vi "ColorTracking_lab.vi"(0 "ROI Descriptor (Color Location 1)":T2={"Global Rectangle"=[20, 20, 620, 460], "Contours"=[{"ID"=enum."External", "Type"=12, "Coordinates"=[20, 20, 620, 460, 0]}]} {"Contours"."Type" items=["No Selection", "Point", "Line", "Rectangle", "Oval", "Polygon", "Freehand Region", "Annulus", "Unused2", "Unused3", "Broken Line", "Freehand Line", "Rotated Rectangle"]}, 1 "File Path (Color Location 1)":path=path "C:/Users/canlasd/Downloads/Labview/Templates/T1.png", 2 "Minimum Match Score (Color Location 1)":sgl=500.0) -> (20 "Matches (Color Location 1)":T3(array[cluster]) {"Bounding Box"."y" format="%.2f"; "Bounding Box"."x" format="%.2f"; "Position"."y" format="%.2f"; "Position"."x" format="%.2f"; "Score" format="%.2f"; "Scale" format="%.2f"; "Angle" format="%.2f"}, 21 "Matches (calibrated) (Color Location 1)":T3(array[cluster]) {"Bounding Box"."y" format="%.2f"; "Bounding Box"."x" format="%.2f"; "Position"."y" format="%.2f"; "Position"."x" format="%.2f"; "Score" format="%.2f"; "Scale" format="%.2f"; "Angle" format="%.2f"}, 22 "Number of Matches (Color Location 1)":i32, 27 "error out":errorcluster)   [LabVIEW 2015]
uses:
  <vilib>/vision/driver/NI_Vision_Acquisition_Software.lvlib
  <vilib>/vision/NI_Vision_Development_Module.lvlib
  <resource>/objmgr/imaqdx.rc
panel:
  in  "Camera Name":refnum<k21> caption="IMAQdx Session"
  in  "Video Modes":i32(listbox)
  in  "Stop":bool
  out "Image":T1(plugin-control)
  out "Buffer Number":u32
  out "Frame Rate":dbl(knob) scale=0.0..100.0
  out "Image Out":T1(plugin-control)
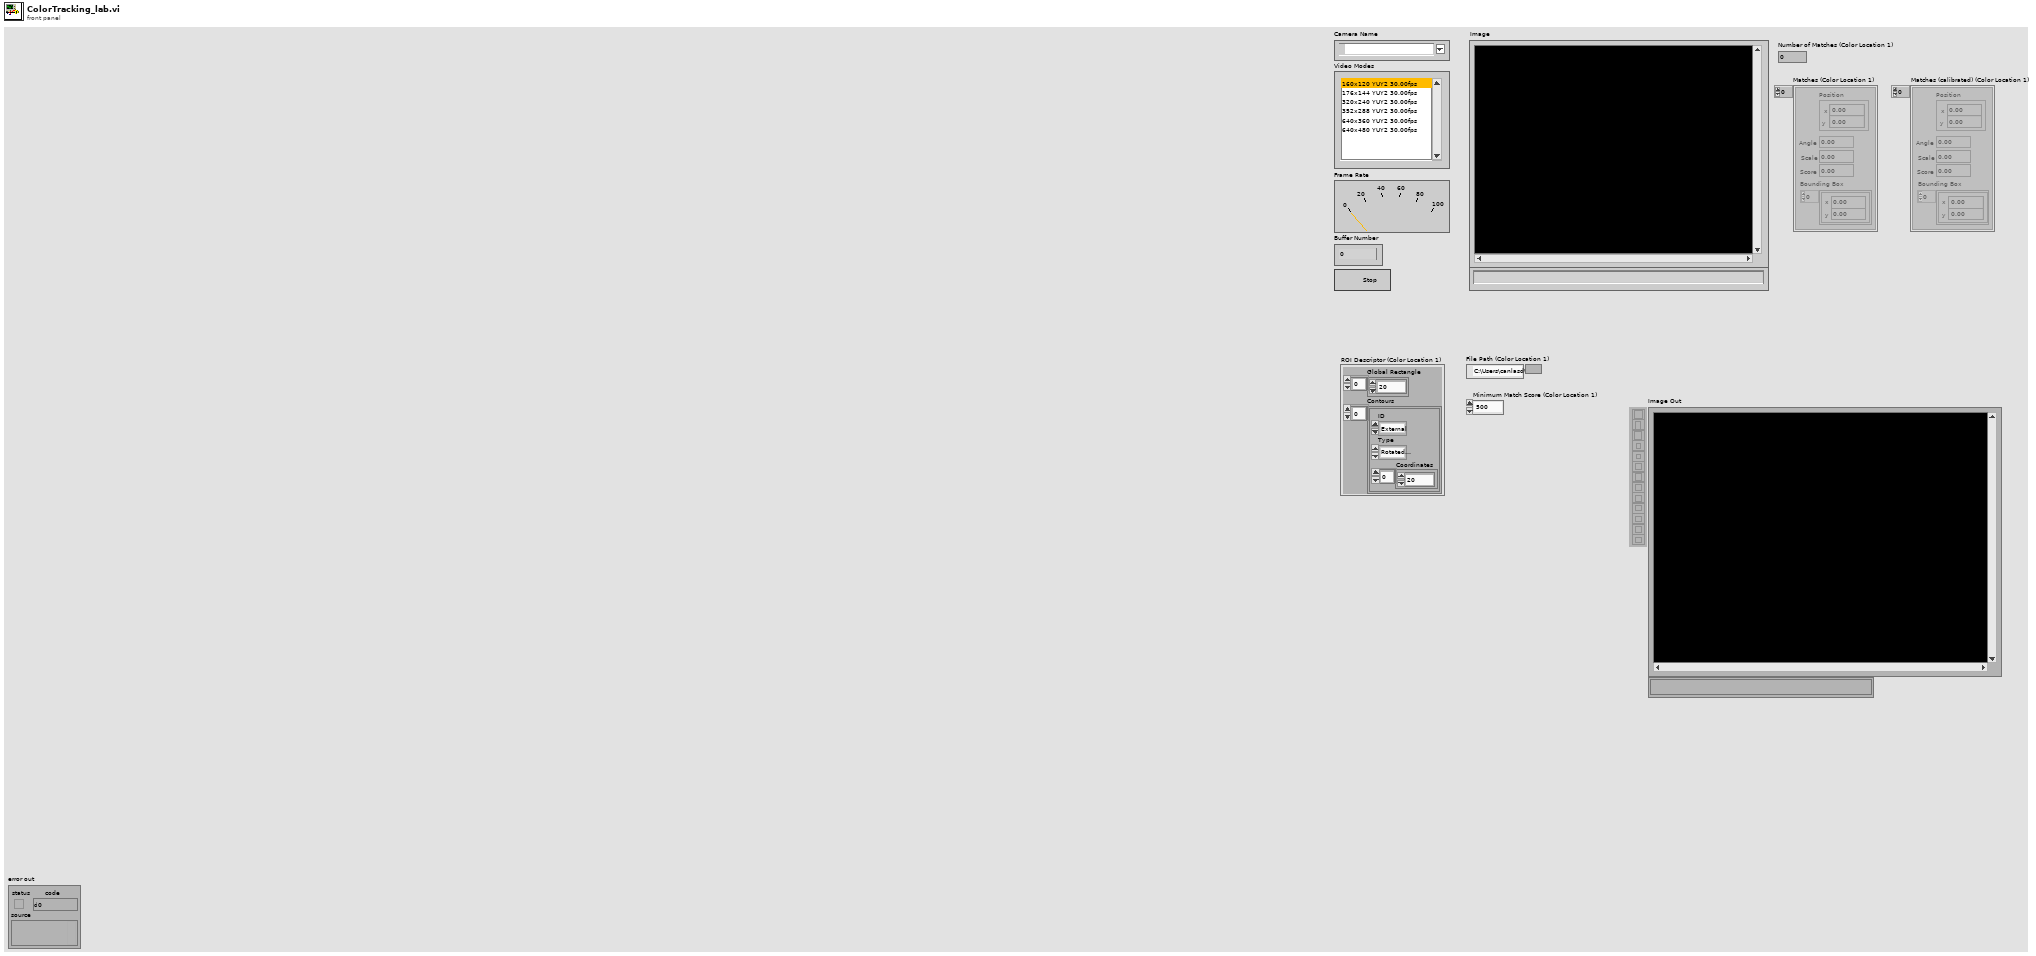
[diagram p1: front panel]
types:
  T1 = typedef "IMAQ Image.ctl" = refnum<image>
  T2 = cluster{"Global Rectangle":i32[], "Contours":cluster{"ID":enum32{"External", "Internal"}, "Type":u32, "Coordinates":i32[]}[]}
  T3 = cluster{"Position":cluster{"x":sgl, "y":sgl}, "Angle":sgl, "Scale":sgl, "Score":sgl, "Bounding Box":cluster{"x":sgl, "y":sgl}[]}[]
  T4 = typedef "IMAQdx.ctl" = refnum<k21>
  T5 = typedef "Image Type" = u32
  T6 = cluster{"Matches[0]":cluster{"Position":cluster{"x":sgl, "y":sgl}, "Angle":sgl, "Scale":sgl, "Score":sgl, "Bounding Box":cluster{"x":sgl, "y":sgl}[]}, "Matches[1]":cluster{"Position":cluster{"x":sgl, "y":sgl}, "Angle":sgl, "Scale":sgl, "Score":sgl, "Bounding Box":cluster{"x":sgl, "y":sgl}[]}, "Matches[2]":cluster{"Position":cluster{"x":sgl, "y":sgl}, "Angle":sgl, "Scale":sgl, "Score":sgl, "Bounding Box":cluster{"x":sgl, "y":sgl}[]}, "Matches[3]":cluster{"Position":cluster{"x":sgl, "y":sgl}, "Angle":sgl, "Scale":sgl, "Score":sgl, "Bounding Box":cluster{"x":sgl, "y":sgl}[]}, "Matches[4]":cluster{"Position":cluster{"x":sgl, "y":sgl}, "Angle":sgl, "Scale":sgl, "Score":sgl, "Bounding Box":cluster{"x":sgl, "y":sgl}[]}, "Matches[5]":cluster{"Position":cluster{"x":sgl, "y":sgl}, "Angle":sgl, "Scale":sgl, "Score":sgl, "Bounding Box":cluster{"x":sgl, "y":sgl}[]}, "Matches[6]":cluster{"Position":cluster{"x":sgl, "y":sgl}, "Angle":sgl, "Scale":sgl, "Score":sgl, "Bounding Box":cluster{"x":sgl, "y":sgl}[]}, "Matches[7]":cluster{"Position":cluster{"x":sgl, "y":sgl}, "Angle":sgl, "Scale":sgl, "Score":sgl, "Bounding Box":cluster{"x":sgl, "y":sgl}[]}, "Matches[8]":cluster{"Position":cluster{"x":sgl, "y":sgl}, "Angle":sgl, "Scale":sgl, "Score":sgl, "Bounding Box":cluster{"x":sgl, "y":sgl}[]}}
  T7 = cluster{"Position":cluster{"x":sgl, "y":sgl}, "Angle":sgl, "Scale":sgl, "Score":sgl, "Bounding Box":cluster{"x":sgl, "y":sgl}[]}
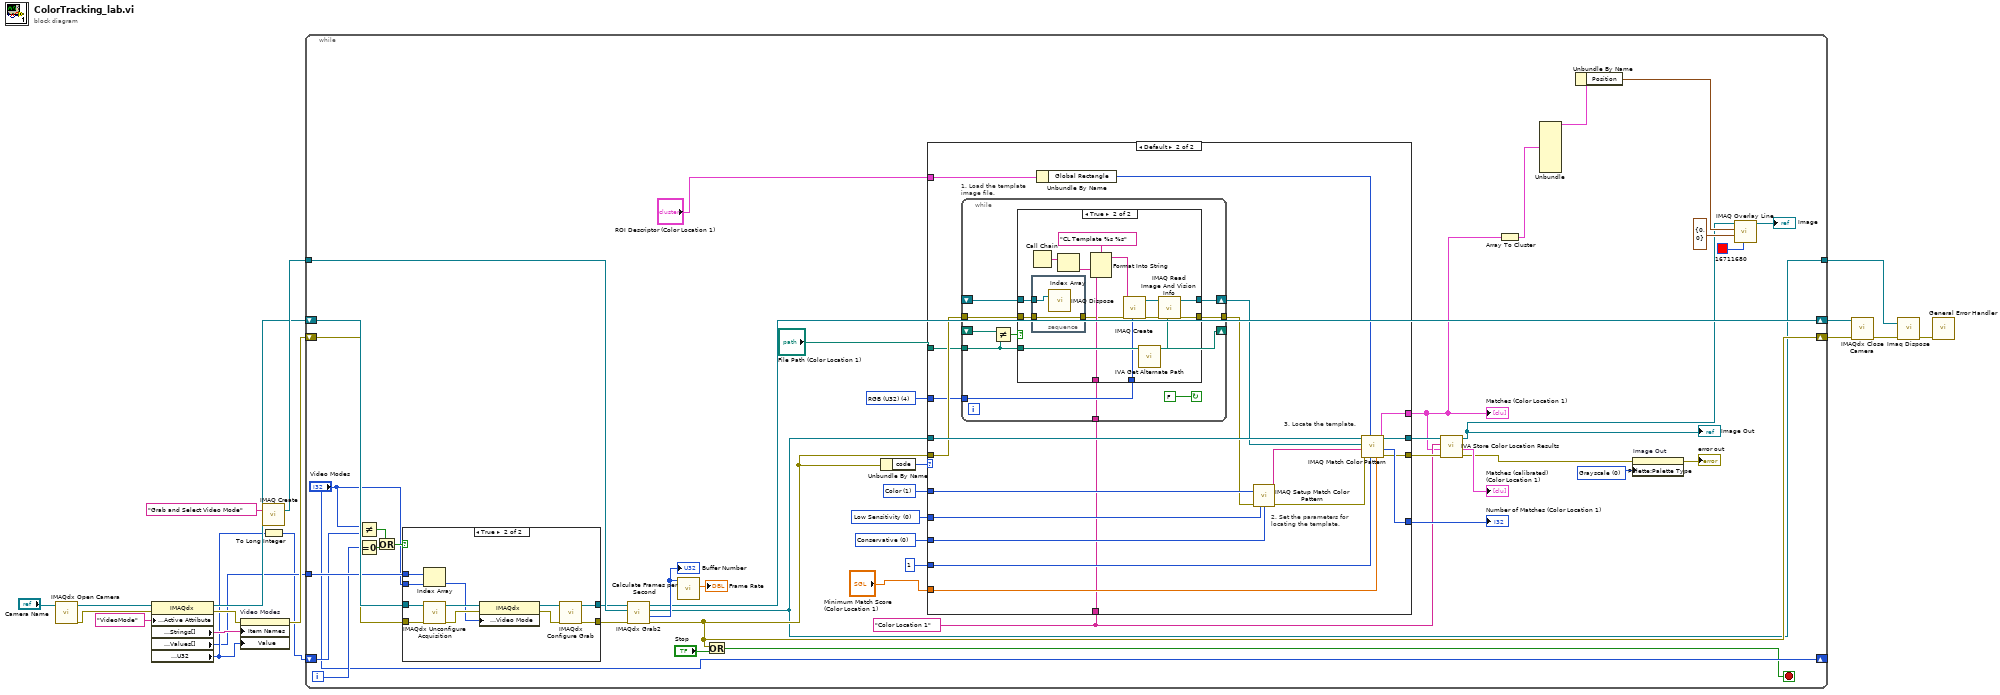
[diagram p0: block diagram]
diagram:
  n1 = call <vilib>:"IMAQdx Open Camera.vi"("Session In"="Camera Name") -> ("error out"=w11:errorcluster, "Session Out"=w13:T4)  [unwired: 2 in, 7 out]
  n2 = property class="IMAQdx"(reference=w13, error in=w11, "Camera Attributes:Active Attribute"="VideoMode" ("ActiveAttribute")) -> (reference out=w9:T4, error out=w10:errorcluster, "Camera Attributes:Enum:Strings[]"=w7:string[], "Camera Attributes:Enum:Values[]"=w2:u32[], "Camera Attributes:Value:U32"=w6:u32)
  n3 = property on="Video Modes" class="LstBox (strict)"(error in=w10, "Item Names"=w7, "Value"=w6) -> (error out=w8:errorcluster)  [unwired: 1 in, 1 out]
  n4 = call "IMAQ Create"("Image Name"="Grab and Select Video Mode") -> ("New Image"=w16:T1)  [unwired: 3 in, 2 out]
  n5 = To Long Integer(number=w6) -> (32bit integer=w1:i32)
  n6 = while {
    tunnel: w2 -> [w42]
    shift-right: [w33] -> w15
    shift-left: w9 -> [w44]
    shift-right: [w29] -> w18
    shift-left: w8 -> [w43]
    tunnel: w16 -> [w45]
    tunnel: [w28] -> w5
    shift-right: ["Video Modes"] -> _
    shift-left: w1 -> [w32]
    i -> [w31]
    stop <- w27 stop-if-true
    w47 = u32 0 items=["Grayscale", "Binary", "Gradient", "Rainbow", "Temperature", "User Defined", "Binary 16 Bit", "Gradient 16 Bit", "Rainbow 16 Bit", "Temperature 16 Bit", "User Defined 16 Bit"] ("Palette Type")
    w49 = "Color Location 1" ("Step Name")
    w56 = T5 4 items=["Grayscale (U8)", "Grayscale (I16)", "Grayscale (SGL)", "Complex (CSG)", "RGB (U32)", "HSL (U32)", "RGB (U64)"] ("Image Type")
    w57 = u32 0 items=["Conservative", "Balance", "Aggressive", "Very Aggressive"] ("Search Strategy")
    w58 = u32 0 items=["Low Sensitivity", "Medium Sensitivity", "High Sensitivity"] ("Color Sensitivity")
    w59 = u32 1 items=["Color and Shape", "Color", "Shape"] ("Match Feature Mode")
    n7 = Not Equal?(x="Video Modes", y=w32) -> (x != y?=w39:bool)
    n8 = Equal To 0?(x=w31) -> (x = 0?=w38:bool)
    n9 = Or(x=w39, y=w38) -> (x .or. y?=w40:bool)
    n10 = case shown="True" w40 {
      tunnel: w44 -> [w64 w73]
      tunnel: w43 -> [w63 w72]
      tunnel: [w64 w69] -> w36
      tunnel: [w63 w70] -> w37
      tunnel: w42 -> [_ w75]
      tunnel: "Video Modes" -> [_ w74]
      frame False {
      }
      frame True {
        n11 = Index Array(array=w75, index=w74) -> (element=w65:u32)
        n12 = call <vilib>:"IMAQdx Unconfigure Acquisition.vi"("error in"=w72, "Session In"=w73) -> ("error out"=w66:errorcluster, "Session Out"=w71:T4)  [unwired: 8 out]
        n13 = property class="IMAQdx"(reference=w71, error in=w66, "Acquisition Attributes:Video Mode"=w65) -> (reference out=w68:T4, error out=w67:errorcluster)
        n14 = call <vilib>:"IMAQdx Configure Grab.vi"("error in"=w67, "Session In"=w68) -> ("error out"=w70:errorcluster, "Session Out"=w69:T4)  [unwired: 1 in, 7 out]
      }
    }
    n15 = call <vilib>:"IMAQdx Grab2.vi"("error in"=w37, "Image In"=w45, "Session In"=w36) -> ("error out"=w29:errorcluster, "Buffer Number Out"=w34:u32, "Image Out"=w28:T1, "Session Out"=w33:T4)  [unwired: 5 in]
    "Buffer Number" <- w34
    n16 = call <vilib>:"Calculate Frames per Second.vi"("Buffer Number"=w34) -> ("Processed Frames/s"=→"Frame Rate":dbl)  [unwired: 8 in, 2 out]
    n17 = Or(x=w29, y="Stop") -> (x .or. y?=w27:bool)
    n18 = Unbundle By Name(w29) -> ("code"=w54:i32)
    n19 = case shown="Default" w54 {
      tunnel: "Minimum Match Score (Color Location 1)" -> [_ w95]
      tunnel: 1 ("Number of Matches Requested") -> [_ w94]
      tunnel: [_ w93] -> w60
      tunnel: w59 -> [_ w92]
      tunnel: w58 -> [_ w91]
      tunnel: w57 -> [_ w90]
      tunnel: "File Path (Color Location 1)" -> [_ w82]
      tunnel: w56 -> [_ w81]
      tunnel: w29 -> [_ w83]
      tunnel: "ROI Descriptor (Color Location 1)" -> [_ w87]
      tunnel: [_ w85] -> w26
      tunnel: w28 -> [w76 w84]
      tunnel: [w76 w84] -> w50
      tunnel: [_ w78] -> w51
      tunnel: w49 -> [_ w77]
      frame -1074396199, -1074396198 {
        # "Discard Coordinate System Error"
      }
      frame Default {
        # "3. Locate the template."
        # "2. Set the parameters for\nlocating the template."
        n20 = while "1. Load the template image file." {
          shift-right: [w105] -> w80
          shift-left: _ -> [w104]
          tunnel: [w102] -> w79
          tunnel: w83 -> [w101]
          tunnel: w82 -> [w96]
          tunnel: w81 -> [w100]
          tunnel: w77 -> [w99]
          shift-right: [w96] -> _
          shift-left: _ -> [w98]
          stop <- FALSE continue-if-true
          n21 = Not Equal?(x=w98, y=w96) -> (x != y?=w97:bool)
          n22 = case shown="True" w97 {
            tunnel: [w107 w120] -> w105
            tunnel: w104 -> [w107 w112]
            tunnel: [w106 w117] -> w102
            tunnel: w101 -> [w106 w111]
            tunnel: w100 -> [_ w116]
            tunnel: w99 -> [_ w113]
            tunnel: w96 -> [_ w109]
            frame False {
            }
            frame True {
              n23 = Call Chain() -> (call chain=w115:string[])
              n24 = stacked-sequence {
                tunnel: w112 -> [w124]
                tunnel: w111 -> [w123]
                tunnel: [w123] -> w110
                frame #0 {
                  n25 = call "IMAQ Dispose"("Image"=w124) -> ()  [unwired: 2 in, 4 out]
                }
              }
              n26 = Index Array(array=w115) -> (element=w114:string)  [unwired: 1 in]
              n27 = Format Into String(format string="CL Template %s %s" ("Image Name"), w114, w113) -> (resulting string=w122:string)  [unwired: 2 in, 1 out]
              n28 = call "IMAQ Create"("Image Name"=w122, "Image Type"=w116, "error in (no error)"=w110) -> ("New Image"=w119:T1, "error out"=w118:errorcluster)  [unwired: 1 in, 1 out]
              n29 = call <vilib>:"IVA Get Alternate Path.vi"("Path In"=w109) -> ("Path Out"=w108:path)  [unwired: 10 out]
              n30 = call "IMAQ Read Image And Vision Info"("File Path"=w108, "error in (no error)"=w118, "Image"=w119) -> ("error out"=w117:errorcluster, "Image Out"=w120:T1)  [unwired: 1 in, 6 out]
            }
          }
        }
        n31 = Unbundle By Name(w87) -> ("Global Rectangle"=w86:i32[])
        n32 = call "IMAQ Setup Match Color Pattern"("Match Feature Mode"=w92, "error in (no error)"=w79, "Color Sensitivity"=w91, "Search Strategy"=w90) -> ("Match Color Pattern Setup Data"=w89:string, "error out"=w88:errorcluster)  [unwired: 5 in, 5 out]
        n33 = call "IMAQ Match Color Pattern"("Minimum Match Score"=w95, "Number of Matches Requested"=w94, "Optional Rectangle"=w86, "error in (no error)"=w88, "Match Color Pattern Setup Data"=w89, "Template Image"=w80, "Image"=w84) -> ("error out"=w78:errorcluster, "Number of Matches"=w93:i32, "Matches"=w85:T3)  [unwired: 2 out]
      }
    }
    "Number of Matches (Color Location 1)" <- w60
    "Matches (Color Location 1)" <- w26
    n34 = call <vilib>:"IVA Store Color Location Results.vi"("error in (no error)"=w51, "Matches"=w26, "Step Name"=w49, "Image in"=w50) -> ("error out"=w52:errorcluster, "Calibrated Matches"=→"Matches (calibrated) (Color Location 1)":T3, "Image dup"=w22:T1)  [unwired: 5 out]
    "Image Out" <- w22
    n35 = Array To Cluster(array=w26) -> (cluster=w25:T6)
    n36 = Unbundle(w25) -> ("Matches[0]"=w19:T7)  [unwired: 8 out]
    n37 = Unbundle By Name "Unbundle By Name"(w19) -> ("Position"=w23:cluster{"x":sgl, "y":sgl})
    n38 = property on="Image Out" class="ImageControl"(error in=w52, "Palette:Palette Type"=w47) -> (error out=→"error out":errorcluster)  [unwired: 1 in, 1 out]
    n39 = call "IMAQ Overlay Line"("Color"=u32 16711680, "End Point"=cluster{"X":i32, "Y":i32} {"X"=0, "Y"=0}, "Start Point"=w23, "Image"=w22) -> ("Image Out"=→"Image":T1)  [unwired: 6 in, 1 out]
  }
  n40 = call <vilib>:"IMAQdx Close Camera.vi"("error in"=w18, "Session In"=w15) -> ("error out"=w4:errorcluster)  [unwired: 9 out]
  n41 = call "Imaq Dispose"("Image"=w5, "error in (no error)"=w4) -> ("error out"=w3:errorcluster)  [unwired: 4 in]
  n42 = call <vilib>:"General Error Handler.vi"("error in (no error)"=w3) -> ()  [unwired: 2 in, 13 out]
